vi "Set Permanent SysEnvVariable.vi"(8 "error in (no error)":errorcluster, 11 "Value":string) -> (0 "error out":errorcluster, 3 "standard output":string)   [LabVIEW 2017]
panel:
  in  "Key":string
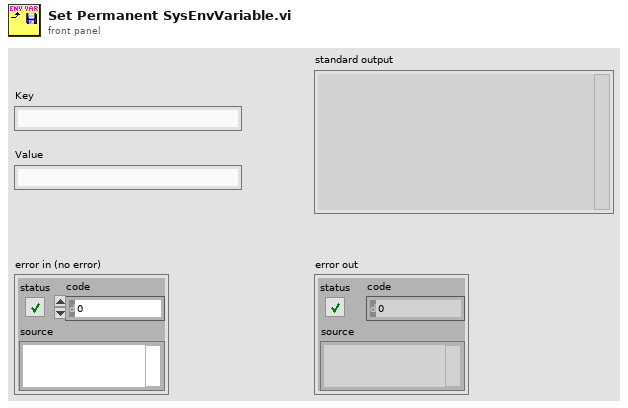
[diagram p1: front panel]
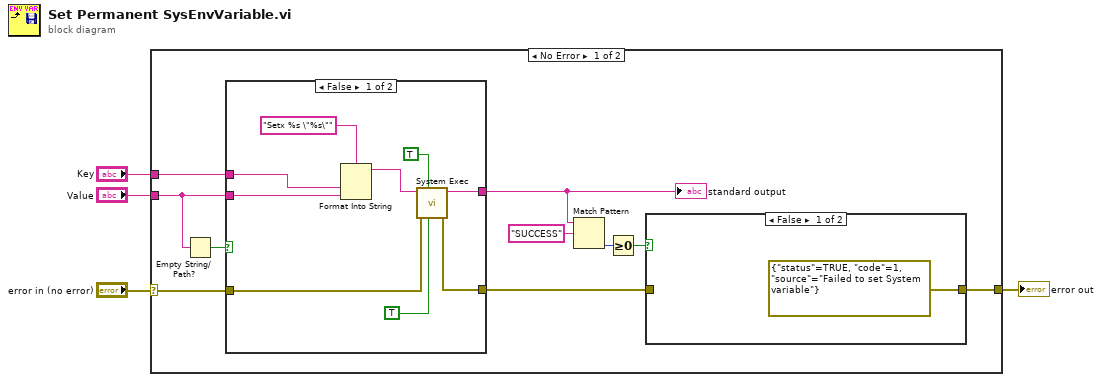
[diagram p0: block diagram]
diagram:
  n1 = case shown="No Error" "error in (no error)" {
    selector: "error in (no error)" -> [w14 w27]
    tunnel: "Value" -> [w11 _]
    tunnel: [w6 w27] -> w2
    tunnel: "Key" -> [w5 _]
    frame No Error {
      n2 = Empty String/Path?(string/path=w11) -> (empty?=w10:bool)
      n3 = case shown="False" w10 {
        tunnel: w14 -> [w25 w26]
        tunnel: [w24 w26] -> w9
        tunnel: [w23 _] -> w13
        tunnel: w11 -> [w21 _]
        tunnel: w5 -> [w20 _]
        frame False {
          n4 = Format Into String(format string="Setx %s \"%s\"" ("string"), w20, w21) -> (resulting string=w19:string)  [unwired: 2 in, 1 out]
          n5 = call <vilib>:"System Exec.vi"("run minimized? (F)"=TRUE, "wait until completion? (T)"=TRUE, "error in (no error)"=w25, "command line"=w19) -> ("error out"=w24:errorcluster, "standard output"=w23:string)  [unwired: 4 in, 2 out]
        }
        frame True {
        }
      }
      "standard output" <- w13
      n6 = Match Pattern(string=w13, regular expression="SUCCESS") -> (offset past match=w8:i32)  [unwired: 1 in, 3 out]
      n7 = Greater Or Equal To 0?(x=w8) -> (x >= 0?=w7:bool)
      n8 = case shown="False" w7 {
        tunnel: w9 -> [_ w16]
        tunnel: [errorcluster {"status"=TRUE, "code"=1, "source"="Failed to set System variable"} ("error IO") w16] -> w6
        frame False {
        }
        frame True {
        }
      }
    }
    frame Error {
    }
  }
  "error out" <- w2
